vi "_API_BINANCE_GET_USDT_FUTURES_Give_amount_of_wallet.vi"(0 "BinanceAPI in":refnum<class "BinanceAPI_.lvclass">, 1 "Isolated %  of  wallet":ext format="%#_3f", 5 "amountOfWallet":cluster{"symbol (eg. BTCUSDT)":string}, 9 "usdt YOU wanna invest":ext format="%#_3f", 11 "error in (no error)":errorcluster) -> (4 "BinanceAPI out":refnum<class "BinanceAPI_.lvclass">, 10 "USDT in crypto (quantity you choose)":ext, 12 "USDT in wallet (avaiable to transaction)":ext, 13 "% USDT from your wallet":ext, 14 "% USDT in crypto in your wallet":ext, 15 "error out":errorcluster)   [LabVIEW 2022 SP3, in "BinanceAPI_.lvclass"]
doc: "Additional Program\n\nFew information from wallet"
uses:
  BinanceAPI_.lvclass
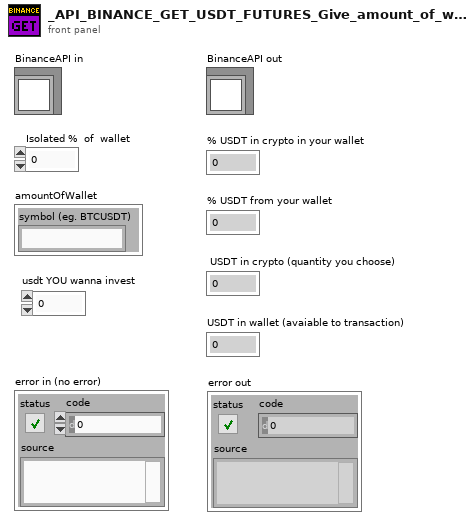
[diagram p1: front panel]
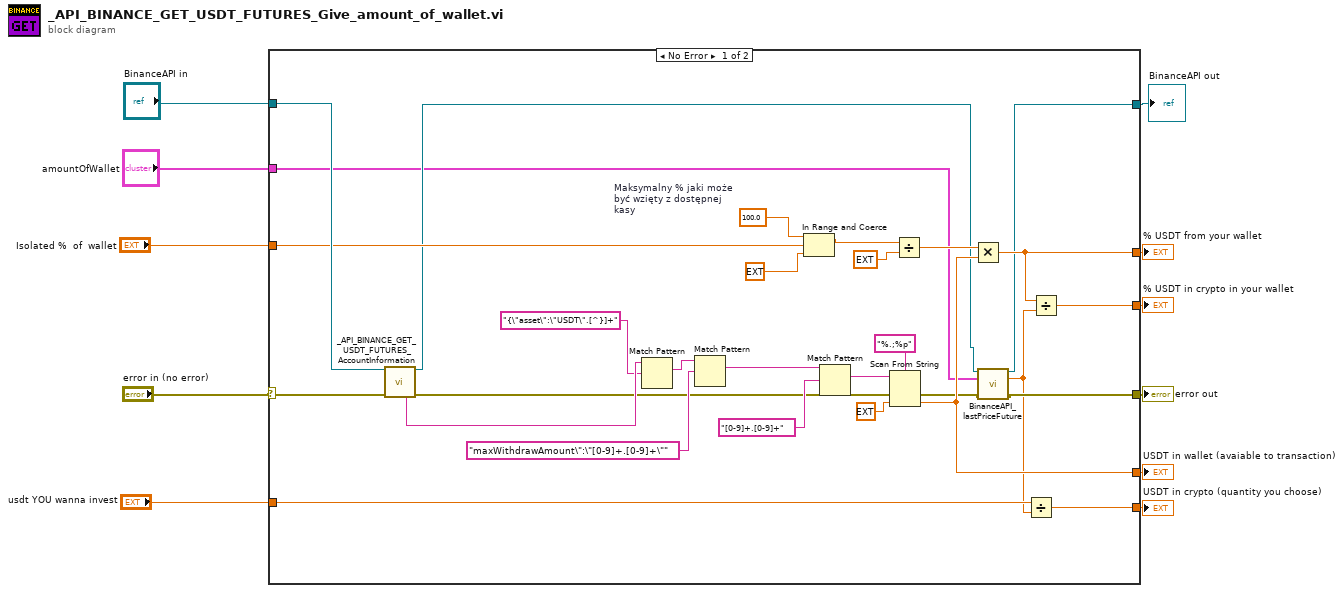
[diagram p0: block diagram]
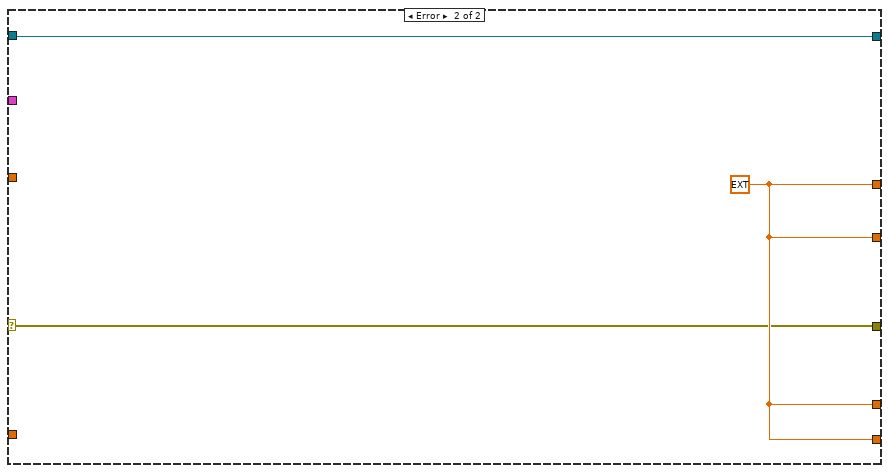
[diagram p2: hidden frame]
diagram:
  n1 = case shown="No Error" "error in (no error)" {
    selector: "error in (no error)" -> [w19 w41]
    tunnel: "BinanceAPI in" -> [w40 w42]
    tunnel: [w18 w43] -> w11
    tunnel: [w14 w41] -> w10
    tunnel: [w32 w43] -> w9
    tunnel: [w31 w43] -> w8
    tunnel: "Isolated %  of  wallet" -> [w25 _]
    tunnel: "amountOfWallet" -> [w13 _]
    tunnel: [w16 w42] -> w2
    tunnel: "usdt YOU wanna invest" -> [w21 _]
    tunnel: [w20 w43] -> w5
    frame No Error {
      w23 = 100.0  # Maksymalny % jaki może być wzięty z dostępnej kasy
      n2 = call "_API_BINANCE_GET_USDT_FUTURES_AccountInformation.vi"("BinanceAPI in"=w40, "error in (no error)"=w19) -> ("BinanceAPI out"=w17:refnum<class "BinanceAPI_.lvclass">, "Data"=w38:string, "error out"=w26:errorcluster)  [unwired: 10 in, 1 out]
      n3 = Match Pattern(string=w38, regular expression="{\"asset\":\"USDT\".[^}]+") -> (match substring=w28:string)  [unwired: 1 in, 3 out]
      n4 = Match Pattern(string=w28, regular expression="maxWithdrawAmount\":\"[0-9]+.[0-9]+\"") -> (match substring=w27:string)  [unwired: 1 in, 3 out]
      n5 = In Range and Coerce(upper limit=w23, x=w25, lower limit=ext 0.0 ("t")) -> (coerced(x)=w24:ext)  [unwired: 1 out]
      n6 = Match Pattern(string=w27, regular expression="[0-9]+.[0-9]+") -> (match substring=w35:string)  [unwired: 1 in, 3 out]
      n7 = Scan From String(format string="%.;%p", input string=w35, error in=w26, default 1=ext 0.0 ("default value 1")) -> (error out=w15:errorcluster, output 1=w18:ext)  [unwired: 1 in, 2 out]
      n8 = Divide(x=w24, y=ext 100.0) -> (x/y=w33:ext)
      n9 = Multiply(x=w33, y=w18) -> (x*y=w32:ext)
      n10 = call "BinanceAPI_lastPriceFuture.vi"("BinanceAPI in"=w17, "lastPrice"=w13, "error in (no error)"=w15) -> ("BinanceAPI out"=w16:refnum<class "BinanceAPI_.lvclass">, "lastPrice"=w12:ext, "error out"=w14:errorcluster)  [unwired: 10 in]
      n11 = Divide(x=w21, y=w12) -> (x/y=w20:ext)
      n12 = Divide(x=w32, y=w12) -> (x/y=w31:ext)
    }
    frame Error {
      w43 = ext 0.0
    }
  }
  "error out" <- w10
  "% USDT from your wallet" <- w9
  "% USDT in crypto in your wallet" <- w8
  "USDT in wallet (avaiable to transaction)" <- w11
  "USDT in crypto (quantity you choose)" <- w5
  "BinanceAPI out" <- w2
